vi "SLSC Get SLSC name from Custom Device Ref.vi"(8 "error in (no error)":errorcluster, 10 "Slot Number":i32, 11 "Item Ref in":T1 format="%.0x") -> (0 "error out":errorcluster, 2 "SLSC Module Name":string, 3 "Item Ref out":T1 format="%.0x")   [LabVIEW 2017, in "SLSC CD System Explorer.lvlib"]
uses:
  SLSC CD System Explorer.lvlib
  <vilib>/NI Veristand/Custom Device API/Custom Device Item Ref.ctl
  Shared/Constants.vi
  Shared/ALMA_10201-10401_O2SensorSim Shared.lvlib
  <vilib>/NI Veristand/Custom Device API/Custom Device API.lvlib
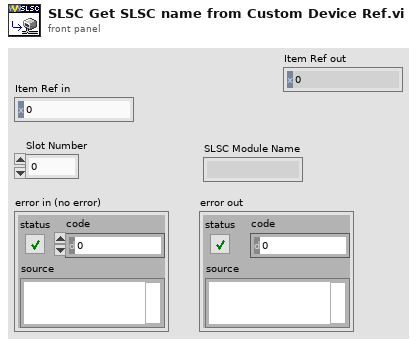
[diagram p1: front panel]
types:
  T1 = typedef "Custom Device API.lvlib/Custom Device Item Ref.ctl" = u64
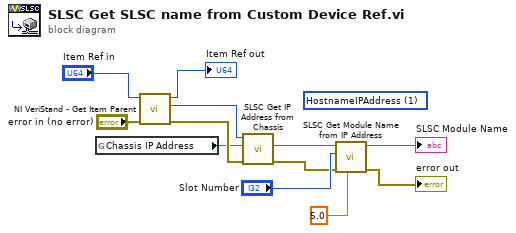
[diagram p0: block diagram]
diagram:
  (unwired) 1 items=["ChassisName", "HostnameIPAddress"] ("Chassis ID Type")
  n1 = global read "Constants.vi" "Chassis IP Address"() -> (w3:string)
  n2 = call <vilib>:"NI VeriStand - Get Item Parent.vi"("error in (no error)"="error in (no error)", "Item Ref in"="Item Ref in") -> ("error out"=w6:errorcluster, "Parent Ref"=w5:T1, "Item Ref out"=→"Item Ref out":T1)  [unwired: 6 in, 1 out]
  n3 = call "SLSC Get IP Address from Chassis.vi"("error in (no error)"=w6, "IP Address Global Name"=w3, "Node Ptr"=w5) -> ("error out"=w10:errorcluster, "Name or IP Address"=w8:string)  [unwired: 3 in, 4 out]
  n4 = call "SLSC Get Module Name from IP Address.vi"("connect timeout"=5.0, "Error In"=w10, "Slot #"="Slot Number", "Chassis IP Address"=w8) -> ("Error Out"=→"error out":errorcluster, "SLSC Module Name"=→"SLSC Module Name":string)  [unwired: 5 in, 1 out]
